vi "Excit_Setup_Wfm_New.vi"(7 "Excit Number":i32, 8 "error in":errorcluster, 9 "Excit Waveforms File Filter":string, 10 "Excit Waveforms Path":path, 11 "Variant":variant) -> (0 "error out":errorcluster caption="sortie d'erreur", 2 "Variant Output":variant, 3 "Waveform Name":string)   [LabVIEW 2015]
doc: "From a start and end value, generates an adiabatic waveform signal of 2000 values (double).\nWrites this waveform into a binary file, in a big-endian format.\nDisplays the written data and the FFT of the signal.\nDefault Path for the generated file is D:\\PIRENEA\\EXCIT_WFMS\n\nAvailable Waveforms : Sinus, Swift, Chirp, Ramp (Up or Down), DoubleRamp (Up-Down or Down-Up)"
uses:
  controls/EXCIT_Waveforms.ctl
  <vilib>/Analysis/NI_AALPro.lvlib
panel:
  in  "EXCIT Waveforms Inputs":T1={"Excit Form"=enum."Swift", "Amplitude"=100.0, "Start Frequency"=250.0, "End Frequency"=1000.0, "Duration"=800.0, "Sampling Frequency"=10.0, "Swift Factor"=0.5, "Chirp Apodisation"=3.5, "Amplitude 2"=100.0, "Start Frequency 2"=250.0, "End Frequency 2"=350.0} {"End Frequency 2" min=1.0 max=10000.0; "Start Frequency 2" min=1.0 max=10000.0; "Amplitude 2" min=1.0 max=100.0; "Chirp Apodisation" min=1.0 max=5.0 step=0.1; "Swift Factor" min=0.1 max=3.0 step=0.1; "Sampling Frequency" min=1.0 max=100.0 step=1.0; "Duration" min=1.0 max=1000000.0 step=1.0; "End Frequency" min=1.0 max=10000.0; "Start Frequency" min=1.0 max=10000.0 step=0.1 format="%#.6g"; "Amplitude" min=1.0 max=100.0}
  out "Waveform Name":string
  in  "OK":bool
  out "Excitation FFT":cluster{dbl[], "Power Spectrum (V^2 rms)":dbl[]}(graph)
  out "Excitation Signal":T2(graph)
  out "FIFO used":i32
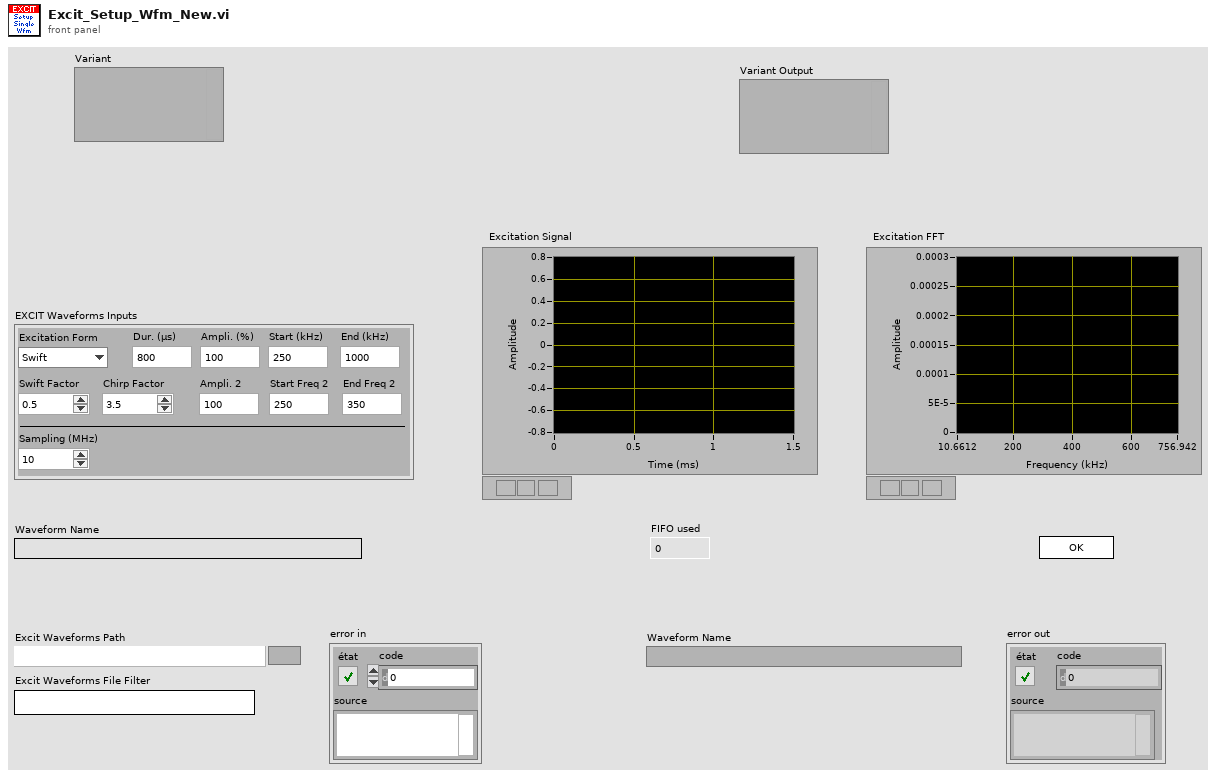
[diagram p1: front panel]
types:
  T1 = typedef "EXCIT_Waveforms.ctl" = cluster{"Excit Form":enum16{"Sinus", "Chirp", "Swift", "TwoSwift", "Ramp"}, "Amplitude":dbl, "Start Frequency":dbl, "End Frequency":dbl, "Duration":dbl, "Sampling Frequency":dbl, "Swift Factor":dbl, "Chirp Apodisation":dbl, "Amplitude 2":dbl, "Start Frequency 2":dbl, "End Frequency 2":dbl}
  T2 = cluster{"X Time":dbl[], "Signal Excitation":dbl[]}
  T3 = enum16{"open", "replace", "create", "open or create", "replace or create", "replace or create with confirmation"}
  T4 = enum16{"big-endian, network order", "native, host order", "little-endian"}
  T5 = enum16{"Sinus", "Chirp", "Swift", "TwoSwift", "Ramp"}
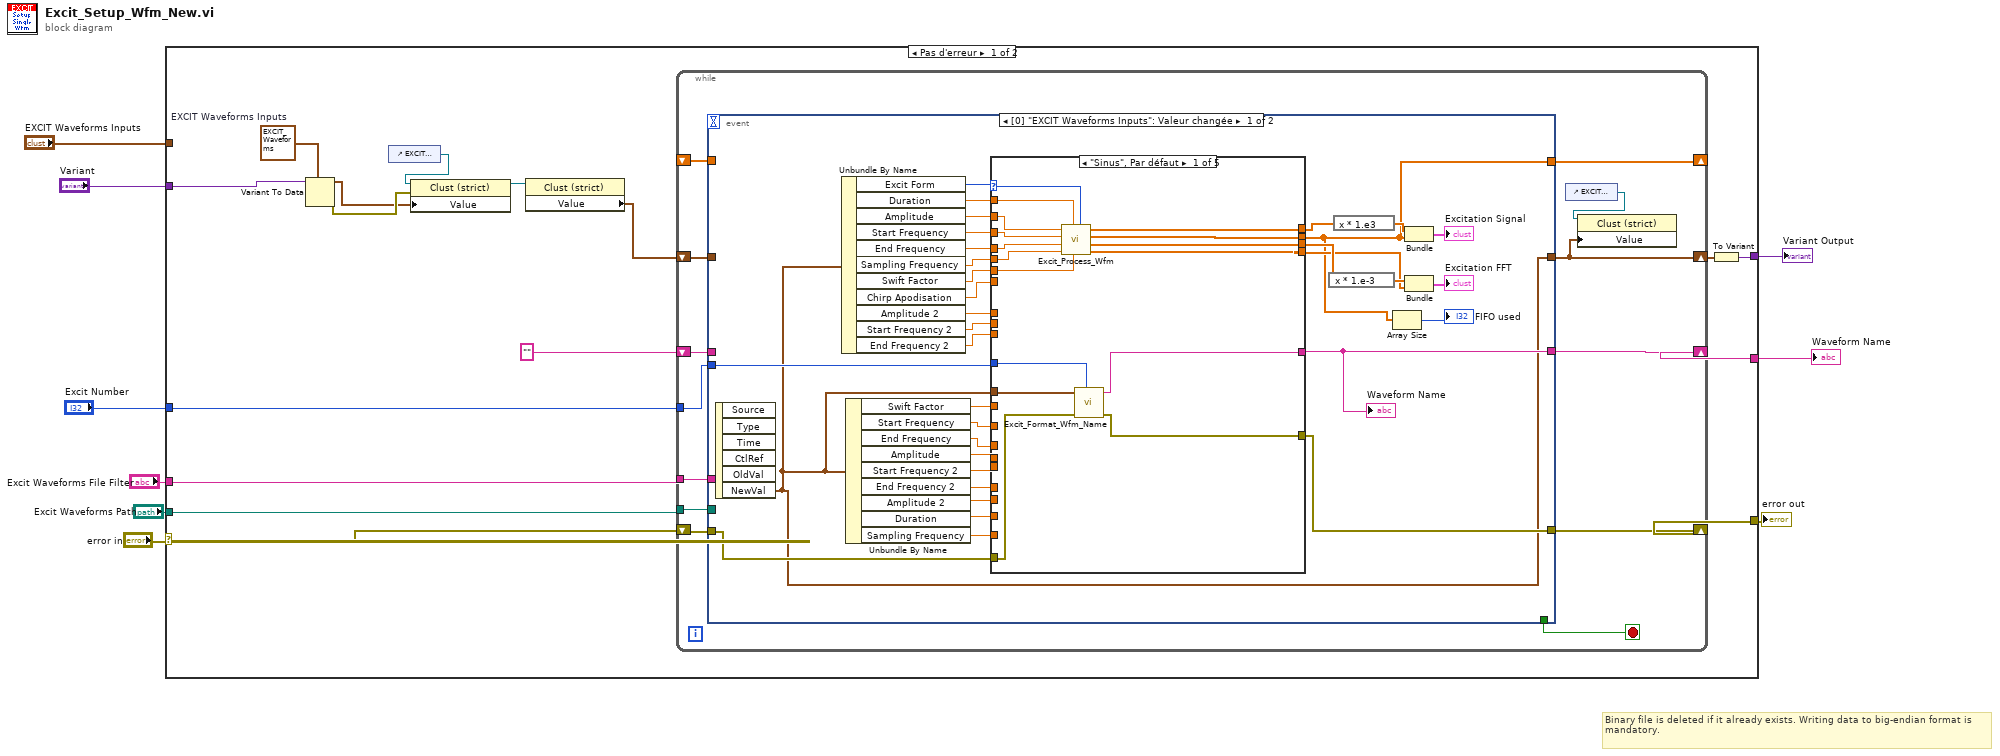
[diagram p0: block diagram]
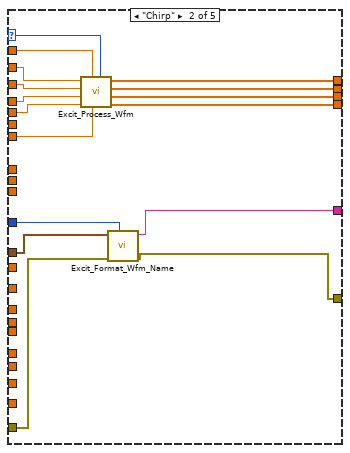
[diagram p2: hidden frame]
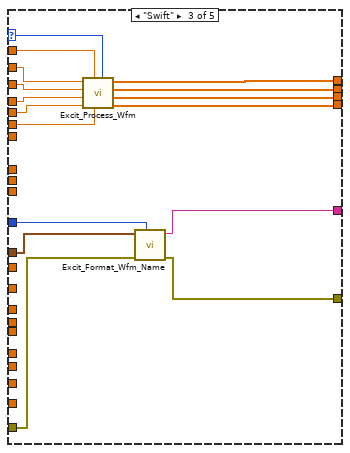
[diagram p3: hidden frame]
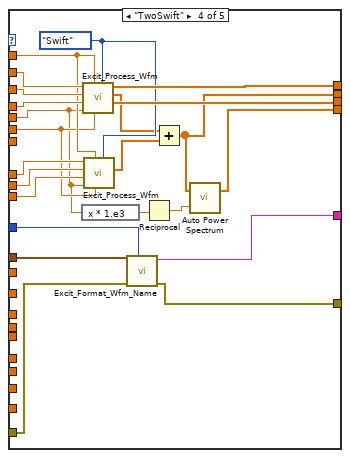
[diagram p4: hidden frame]
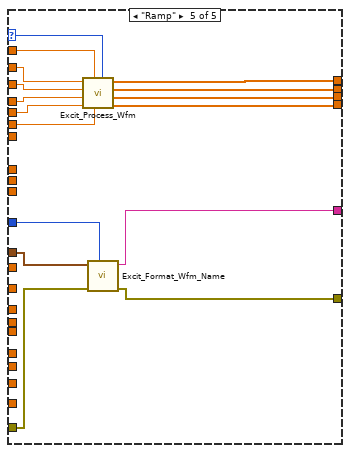
[diagram p5: hidden frame]
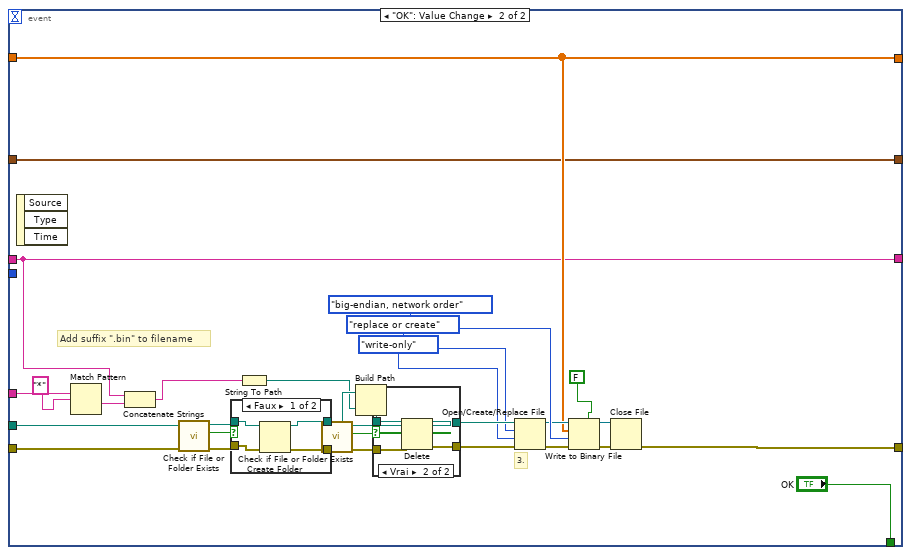
[diagram p6: hidden frame]
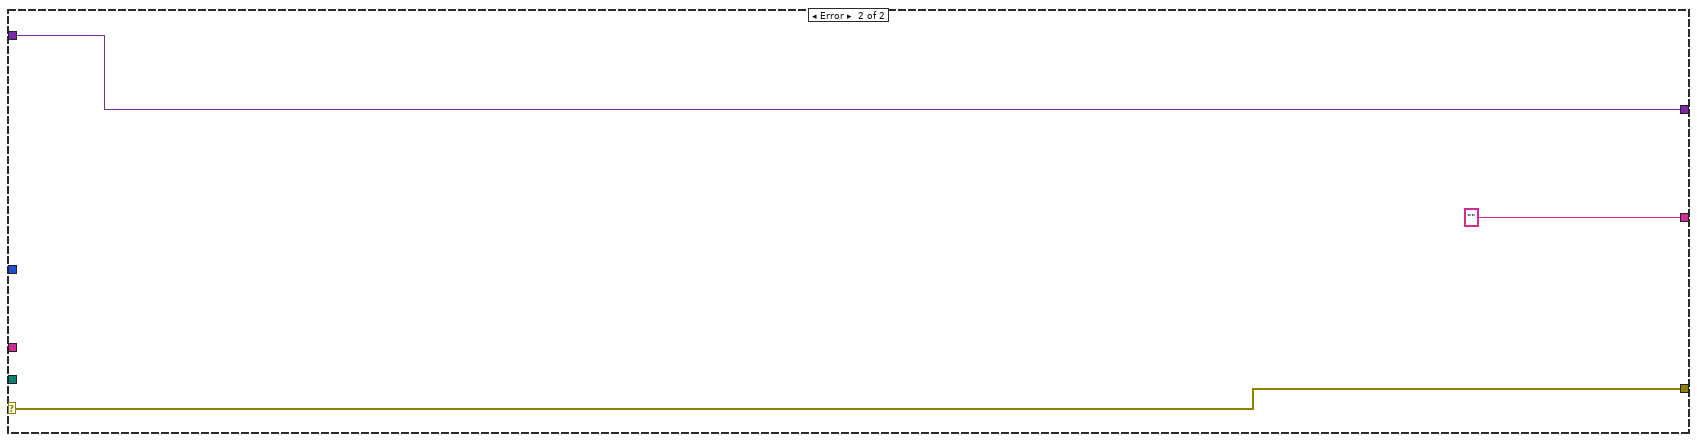
[diagram p9: hidden frame]
diagram:
  # "Binary file is deleted if it already exists. Writing data to big-endian format is mandatory."
  n1 = case shown="Pas d'erreur" "error in" {
    selector: "error in" -> [w20 w205]
    tunnel: [w25 w205] -> w9
    tunnel: "Excit Waveforms Path" -> [w24 _]
    tunnel: [w23 ""] -> w6
    tunnel: "Excit Waveforms File Filter" -> [w22 _]
    tunnel: [w16 w203] -> w2
    tunnel: "Excit Number" -> [w19 _]
    tunnel: "Variant" -> [w18 w203]
    tunnel: "EXCIT Waveforms Inputs" -> [_ _]
    frame No Error {
      w11 = T1 {"Excit Form"=enum."Swift", "Amplitude"=100.0, "Start Frequency"=250.0, "End Frequency"=1000.0, "Duration"=800.0, "Sampling Frequency"=10.0, "Swift Factor"=0.5, "Chirp Apodisation"=3.5, "Amplitude 2"=100.0, "Start Frequency 2"=250.0, "End Frequency 2"=350.0}  # EXCIT Waveforms Inputs
      n2 = Variant To Data(type=w11, Variant=w18) -> (data=w10:T1, error out=w15:errorcluster)  [unwired: 1 in]
      n3 = control-ref of="EXCIT Waveforms Inputs"() -> (w12:refnum<vi>)
      n4 = property class="Clust (strict)"(reference=w12, error in=w15, "Value"=w10) -> (reference out=w14:refnum<vi>)  [unwired: 1 out]
      n5 = property class="Clust (strict)"(reference=w14) -> ("Value"=w13:T1)  [unwired: 1 in, 2 out]
      n6 = while {
        tunnel: w24 -> [w32]
        shift-right: [w31] -> w25
        shift-left: w20 -> [w38]
        shift-right: [w36] -> _
        shift-left: _ -> [w34]
        shift-right: [w35] -> w23
        shift-left: "" -> [w33]
        tunnel: w22 -> [w30]
        shift-right: [w26] -> w17
        shift-left: w13 -> [w28]
        tunnel: w19 -> [w29]
        stop <- w37 stop-if-true
        n7 = event shown="[0] \"EXCIT Waveforms Inputs\": Valeur changée" {
          selector: _ -> [_ _]
          dyn-events: _ -> [_ _]
          timeout: _ -> [_ _]
          tunnel: [w44 w167] -> w31
          tunnel: w38 -> [w46 w169]
          tunnel: [_ "OK"] -> w37
          tunnel: [w45 w166] -> w36
          tunnel: [w43 w162] -> w35
          tunnel: w34 -> [_ w166]
          tunnel: w33 -> [_ w162]
          tunnel: w32 -> [_ w168]
          tunnel: w30 -> [_ w165]
          tunnel: w29 -> [w42 _]
          tunnel: [w39 w160] -> w26
          tunnel: w28 -> [_ w160]
          event Value Change {
            n8 = event-data() -> ("NewVal"=w39:T1)  [unwired: 1 in, 5 out]
            n9 = Unbundle By Name(w39) -> ("Excit Form"=w40:T5, "Duration"=w69:dbl, "Amplitude"=w68:dbl, "Start Frequency"=w67:dbl, "End Frequency"=w66:dbl, "Sampling Frequency"=w65:dbl, "Swift Factor"=w64:dbl, "Chirp Apodisation"=w63:dbl, "Amplitude 2"=w57:dbl, "Start Frequency 2"=w56:dbl, "End Frequency 2"=w55:dbl)
            n10 = Unbundle By Name(w39) -> ("Swift Factor"=w41:dbl, "Start Frequency"=w54:dbl, "End Frequency"=w53:dbl, "Amplitude"=w52:dbl, "Start Frequency 2"=w47:dbl, "End Frequency 2"=w51:dbl, "Amplitude 2"=w50:dbl, "Duration"=w49:dbl, "Sampling Frequency"=w48:dbl)
            n11 = case shown="\"Sinus\", Par défaut" w40 {
              selector: w40 -> [w88 w104 w120 _ w155]
              tunnel: w63 -> [_ w89 _ _ _]
              tunnel: w69 -> [w78 w94 w111 w127 w149]
              tunnel: w68 -> [w77 w93 w110 w130 w148]
              tunnel: w67 -> [w76 w92 w109 w129 w147]
              tunnel: w66 -> [w75 w91 w108 w128 w146]
              tunnel: w65 -> [w74 w90 w107 w122 w145]
              tunnel: w64 -> [w73 _ w106 w123 w144]
              tunnel: [w87 w103 w119 w143 w159] -> w62
              tunnel: [w86 w102 w118 w137 w158] -> w45
              tunnel: [w85 w101 w117 w142 w157] -> w60
              tunnel: [w84 w100 w116 w135 w156] -> w59
              tunnel: w57 -> [_ _ _ w126 _]
              tunnel: w56 -> [_ _ _ w125 _]
              tunnel: w55 -> [_ _ _ w124 _]
              tunnel: [w81 w96 w113 w131 w153] -> w44
              tunnel: [w80 w97 w112 w132 w151] -> w43
              tunnel: w54 -> [_ _ _ _ _]
              tunnel: w53 -> [_ _ _ _ _]
              tunnel: w52 -> [_ _ _ _ _]
              tunnel: w51 -> [_ _ _ _ _]
              tunnel: w50 -> [_ _ _ _ _]
              tunnel: w49 -> [_ _ _ _ _]
              tunnel: w48 -> [_ _ _ _ _]
              tunnel: w47 -> [_ _ _ _ _]
              tunnel: w46 -> [w82 w98 w114 w133 w154]
              tunnel: w42 -> [w83 w99 w115 w134 w152]
              tunnel: w41 -> [_ _ _ _ _]
              tunnel: w39 -> [w79 w95 w105 w121 w150]
              frame "Sinus", Default {
                n12 = call "Excit_Process_Wfm.vi"("Excit Form"=w88, "Factor"=w73, "Duration (µs)"=w78, "Sampling Frequency (MHz)"=w74, "End Frequency (kHz)"=w75, "Start Frequency (kHz)"=w76, "Amplitude (%)"=w77) -> ("FFT Excitation"=w84:dbl[], "X Freq"=w85:dbl[], "Signal Excitation"=w86:dbl[], "X Time"=w87:dbl[])
                n13 = call "Excit_Format_Wfm_Name.vi"("Excit Number"=w83, "error in"=w82, "EXCIT Waveforms Inputs"=w79) -> ("error out"=w81:errorcluster, "Waveform Name"=w80:string)  [unwired: 7 in]
              }
              frame "Chirp" {
                n14 = call "Excit_Process_Wfm.vi"("Excit Form"=w104, "Factor"=w89, "Duration (µs)"=w94, "Sampling Frequency (MHz)"=w90, "End Frequency (kHz)"=w91, "Start Frequency (kHz)"=w92, "Amplitude (%)"=w93) -> ("FFT Excitation"=w100:dbl[], "X Freq"=w101:dbl[], "Signal Excitation"=w102:dbl[], "X Time"=w103:dbl[])
                n15 = call "Excit_Format_Wfm_Name.vi"("Excit Number"=w99, "error in"=w98, "EXCIT Waveforms Inputs"=w95) -> ("error out"=w96:errorcluster, "Waveform Name"=w97:string)  [unwired: 7 in]
              }
              frame "Swift" {
                n16 = call "Excit_Process_Wfm.vi"("Excit Form"=w120, "Factor"=w106, "Duration (µs)"=w111, "Sampling Frequency (MHz)"=w107, "End Frequency (kHz)"=w108, "Start Frequency (kHz)"=w109, "Amplitude (%)"=w110) -> ("FFT Excitation"=w116:dbl[], "X Freq"=w117:dbl[], "Signal Excitation"=w118:dbl[], "X Time"=w119:dbl[])
                n17 = call "Excit_Format_Wfm_Name.vi"("Excit Number"=w115, "error in"=w114, "EXCIT Waveforms Inputs"=w105) -> ("error out"=w113:errorcluster, "Waveform Name"=w112:string)  [unwired: 7 in]
              }
              frame "TwoSwift" {
                w141 = T5."Swift" ("Excit Form")
                n18 = expression code="x * 1.e3"(w122) -> (w138:dbl)
                n19 = call "Excit_Process_Wfm.vi"("Excit Form"=w141, "Factor"=w123, "Duration (µs)"=w127, "Sampling Frequency (MHz)"=w122, "End Frequency (kHz)"=w128, "Start Frequency (kHz)"=w129, "Amplitude (%)"=w130) -> ("X Freq"=w142:dbl[], "Signal Excitation"=w140:dbl[], "X Time"=w143:dbl[])  [unwired: 1 out]
                n20 = call "Excit_Process_Wfm.vi"("Excit Form"=w141, "Factor"=w123, "Duration (µs)"=w127, "Sampling Frequency (MHz)"=w122, "End Frequency (kHz)"=w124, "Start Frequency (kHz)"=w125, "Amplitude (%)"=w126) -> ("Signal Excitation"=w139:dbl[])  [unwired: 3 out]
                n21 = call "Excit_Format_Wfm_Name.vi"("Excit Number"=w134, "error in"=w133, "EXCIT Waveforms Inputs"=w121) -> ("error out"=w131:errorcluster, "Waveform Name"=w132:string)  [unwired: 7 in]
                n22 = Reciprocal(x=w138) -> (1/x=w136:dbl)
                n23 = Add(x=w140, y=w139) -> (x+y=w137:dbl[])
                n24 = call <vilib>:"Auto Power Spectrum.vi"("dt"=w136, "Signal (V)"=w137) -> ("Power Spectrum (V^2 rms)"=w135:dbl[])  [unwired: 1 out]
              }
              frame "Ramp" {
                n25 = call "Excit_Process_Wfm.vi"("Excit Form"=w155, "Factor"=w144, "Duration (µs)"=w149, "Sampling Frequency (MHz)"=w145, "End Frequency (kHz)"=w146, "Start Frequency (kHz)"=w147, "Amplitude (%)"=w148) -> ("FFT Excitation"=w156:dbl[], "X Freq"=w157:dbl[], "Signal Excitation"=w158:dbl[], "X Time"=w159:dbl[])
                n26 = call "Excit_Format_Wfm_Name.vi"("Excit Number"=w152, "error in"=w154, "EXCIT Waveforms Inputs"=w150) -> ("error out"=w153:errorcluster, "Waveform Name"=w151:string)  [unwired: 7 in]
              }
            }
            "Waveform Name" <- w43
            n27 = expression code="x * 1.e-3"(w60) -> (w70:dbl[])
            n28 = expression code="x * 1.e3"(w62) -> (w71:dbl[])
            n29 = Array Size(array=w45) -> (size(s)=→"FIFO used":i32)
            n30 = Bundle("X Time"=w71, "Signal Excitation"=w45) -> (→"Excitation Signal":T2)  [unwired: 1 in]
            n31 = Bundle("X Freq"=w70, "FFT Excitation"=w59) -> (→"Excitation FFT":cluster{"X Freq":dbl[], "FFT Excitation":dbl[]})  [unwired: 1 in]
          }
          event "OK": Value Change {
            # "Add suffix \".bin\" to filename"
            # "3."
            n32 = event-data() -> ()  [unwired: 1 in, 3 out]
            n33 = Match Pattern(string=w165, regular expression="*" ("expression régulière")) -> (after substring=w163:string)  [unwired: 1 in, 3 out]
            n34 = Concatenate Strings(w162, w163) -> (w161:string)
            n35 = call <vilib>:"Check if File or Folder Exists.vi"("error in (no error)"=w169, "path"=w168) -> ("error out"=w187:errorcluster, "file or folder exists?"=w185:bool, "dup path"=w186:path)  [unwired: 7 in]
            n36 = case shown="Faux" w185 {
              tunnel: w186 -> [w194 w196]
              tunnel: [w193 w196] -> w188
              tunnel: w187 -> [w192 w195]
              tunnel: [w191 w195] -> w189
              frame False {
                n37 = Create Folder(path (use dialog)=w194, error in=w192) -> (created path=w193:path, error out=w191:errorcluster)  [unwired: 1 in, 1 out]
              }
              frame True {
              }
            }
            n38 = String To Path(string=w161) -> (path=w178:path)
            n39 = Build Path(base path=w188, name or relative path=w178) -> (appended path=w182:path)
            n40 = call <vilib>:"Check if File or Folder Exists.vi"("error in (no error)"=w189, "path"=w182) -> ("error out"=w181:errorcluster, "file or folder exists?"=w180:bool, "dup path"=w179:path)  [unwired: 7 in]
            n41 = case shown="Vrai" w180 {
              tunnel: w179 -> [w198 w202]
              tunnel: w181 -> [w197 w201]
              tunnel: [w198 w200] -> w183
              tunnel: [w197 w199] -> w184
              frame False {
              }
              frame True {
                n42 = Delete(path (use dialog)=w202, error in=w201) -> (deleted path=w200:path, error out=w199:errorcluster)  [unwired: 3 in, 1 out]
              }
            }
            n43 = Open/Create/Replace File(file path (use dialog)=w183, error in=w184, operation (0:open)=T3."replace or create", access (0:read/write)=enum16{"read/write", "read-only", "write-only"}."write-only") -> (refnum out=w173:refnum<file>, error out=w172:errorcluster)  [unwired: 2 in, 1 out]
            n44 = Write to Binary File(file (use dialog)=w173, data=w166, error in=w172, 5:FALSE ("prepend array or string size? (T)"), 9:T4."big-endian, network order" ("byte order")) -> (refnum out=w170:refnum<file>, error out=w171:errorcluster)  [unwired: 1 in, 1 out]
            n45 = Close File(refnum=w170, error in=w171) -> (error out=w167:errorcluster)  [unwired: 1 out]
          }
        }
        n46 = control-ref of="EXCIT Waveforms Inputs"() -> (w27:refnum<vi>)
        n47 = property class="Clust (strict)"(reference=w27, "Value"=w26) -> ()  [unwired: 1 in, 2 out]
      }
      n48 = To Variant(anything=w17) -> (Variant=w16:variant)
    }
    frame Error {
    }
  }
  "error out" <- w9
  "Waveform Name" <- w6
  "Variant Output" <- w2
